vi "login.vi"() -> ()   [LabVIEW 2017]
panel:
  out "Boolean 2":bool
  out "Boolean":bool
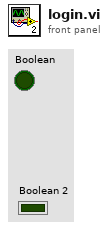
[diagram p1: front panel]
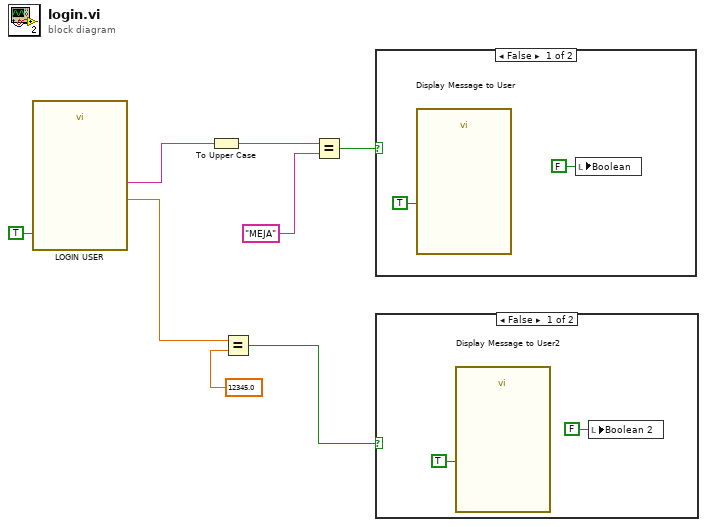
[diagram p0: block diagram]
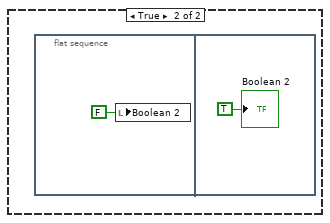
[diagram p2: hidden frame]
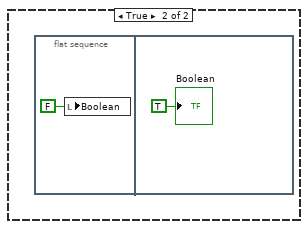
[diagram p3: hidden frame]
diagram:
  n1 = call "LOGIN USER"("Enable"=TRUE) -> ("Badge ID"=w8:dbl, "Login"=w2:string)  [unwired: 15 in, 2 out]
  n2 = To Upper Case(1:w2) -> (0:w1:string)
  n3 = Equal?(x=w8, y=12345.0) -> (x = y?=w5:bool)
  n4 = Equal?(x=w1, y="MEJA") -> (x = y?=w6:bool)
  n5 = case shown="False" w6 {
    frame False {
      n6 = call "Display Message to User"("Enable"=TRUE) -> ()  [unwired: 9 in, 2 out]
      n7 = local write "Boolean"(FALSE ("Boolean")) -> ()
    }
    frame True {
      n8 = flat-sequence {
        frame #0 {
          n9 = local write "Boolean"(FALSE ("Boolean")) -> ()
        }
        frame #1 {
          "Boolean" <- TRUE ("Boolean")
        }
      }
    }
  }
  n10 = case shown="False" w5 {
    frame False {
      n11 = call "Display Message to User2"("Enable"=TRUE) -> ()  [unwired: 9 in, 2 out]
      n12 = local write "Boolean 2"(FALSE ("Boolean 2")) -> ()
    }
    frame True {
      n13 = flat-sequence {
        frame #0 {
          n14 = local write "Boolean 2"(FALSE ("Boolean 2")) -> ()
        }
        frame #1 {
          "Boolean 2" <- TRUE ("Boolean 2")
        }
      }
    }
  }
